vi "Play Path.vi"(7 "Description":string, 8 "Command Info In":T3, 10 "Synchronization":enum16{"Start", "Wait"}(ring), 11 "Auto Data":T1) -> (0 "Command Info Out":T3)   [LabVIEW 2025]
doc: "This VI notifies the subsystem to the new setpoint."
uses:
  Implementation/Drive Operations.ctl
  Implementation/Drive Setpoints.ctl
  swerve-template/Type Definitions/Data/Robot Velocities.ctl
  Framework/Robot Global Data.vi
  Implementation/Auto Data.ctl
  <vilib>/Rock Robotics/WPI/Framework/Completion Status.ctl
  <vilib>/Rock Robotics/WPI/Framework/Completion Notifier.ctl
  <vilib>/Rock Robotics/WPI/Framework/Command Status Info.ctl
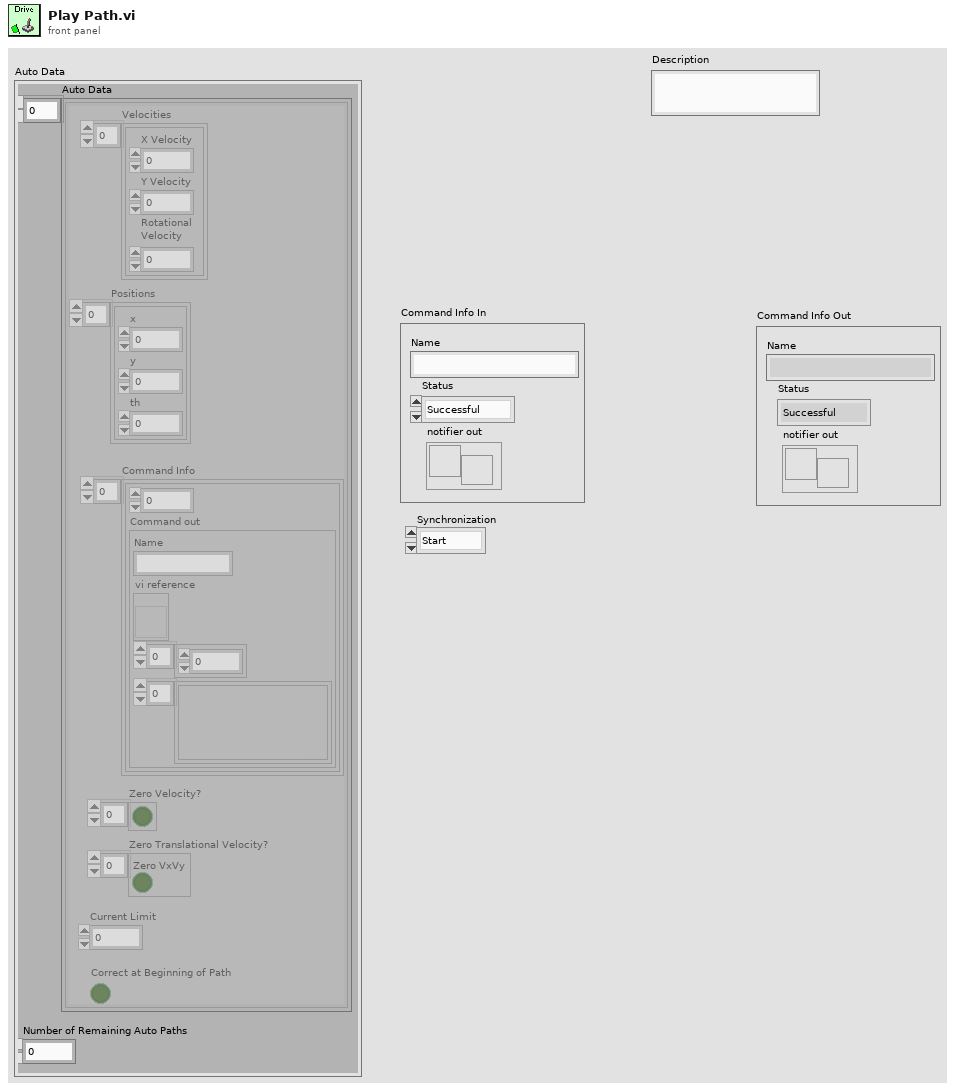
[diagram p1: front panel]
types:
  T1 = typedef "Auto Data.ctl" = cluster{"Auto Data":cluster{"Velocities":T2[], "Positions":cluster{"x":dbl, "y":dbl, "th":dbl}[], "Command Info":cluster{dbl, "Command out":cluster{"Name":string, "vi reference":refnum<vi>, i32[], variant[]}}[], "Zero Velocity?":bool[], "Zero Translational Velocity?":bool[], "Current Limit":dbl, "Correct at Beginning of Path":bool}[], "Number of Remaining Auto Paths":dbl}
  T2 = typedef "Robot Velocities.ctl" = cluster{"X Velocity":dbl, "Y Velocity":dbl, "Rotational \nVelocity":dbl}
  T3 = typedef "Command Status Info.ctl" = cluster{"Name":string, "Status":T4, "notifier out":T5}
  T4 = typedef "Completion Status.ctl" = enum16{"Successful", "Aborted", "Incomplete"}
  T5 = typedef "Completion Notifier.ctl" = refnum<notifier>
  T6 = typedef "Drive Setpoints.ctl" = cluster{"Operation":T7, "Robot Velocities":T2, "Auto Data":T1}
  T7 = typedef "Drive Operations.ctl" = enum16{"Reserve", "Read Current", "Immediate", "Calibrate", "Auto", "Auto Pickup"}
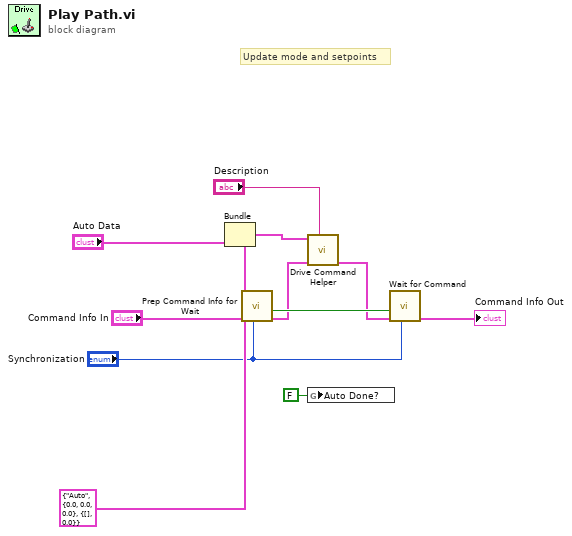
[diagram p0: block diagram]
diagram:
  # "Update mode and setpoints"
  n1 = Bundle(cluster=T6 {"Operation"=enum."Auto", "Robot Velocities"={"X Velocity"=0.0, "Y Velocity"=0.0, "Rotational \nVelocity"=0.0}, "Auto Data"={"Auto Data"=[], "Number of Remaining Auto Paths"=0.0}} ("SubSystem Data"), "Auto Data"="Auto Data") -> (w10:T6)  [unwired: 2 in]
  n2 = call <vilib>:"Prep Command Info for Wait.vi"("Synchronication"="Synchronization", "Command Info"="Command Info In") -> ("Command Info"=w5:T3, "Allocated"=w8:bool)  [unwired: 8 in]
  n3 = call "Drive Command Helper.vi"("Description"="Description", "Command Info In"=w5, "SubSystem Data"=w10) -> ("Command Info Out"=w4:T3)  [unwired: 6 in, 2 out]
  n4 = global write "Robot Global Data.vi" "Auto Done?"(FALSE ("Auto Done?")) -> ()
  n5 = call <vilib>:"Wait for Command.vi"("Synchronication"="Synchronization", "Command Info in"=w4, "Allocated"=w8) -> ("Command Info out"=→"Command Info Out":T3)  [unwired: 8 in]
